vi "Configure Tone.vi"(0 "VISA resource name":refnum<visa-resource-name>, 1 "Frequency (1000 Hz)":dbl=1000.0, 2 "Phase (0 degrees)":dbl, 5 "Tone Channel (0: A)":i32(ring) items=["A", "B"], 7 "Tone Number (0)":i32, 9 "Amplitude (100 %)":dbl=100.0, 11 "error in (no error)":errorcluster, 12 "Enable Tone (T: Enable)":bool=TRUE) -> (4 "VISA resource name out":refnum<visa-resource-name>, 15 "error out":errorcluster)   [LabVIEW 2014, in "Stanford Research SR1.lvlib"]
doc: "Configures the attributes for the Tone."
uses:
  Stanford Research SR1.lvlib
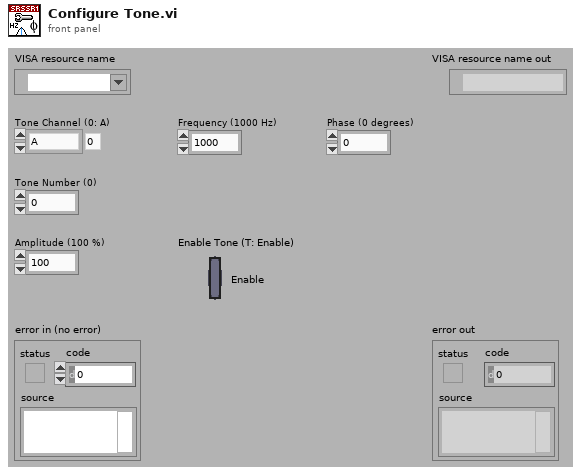
[diagram p1: front panel]
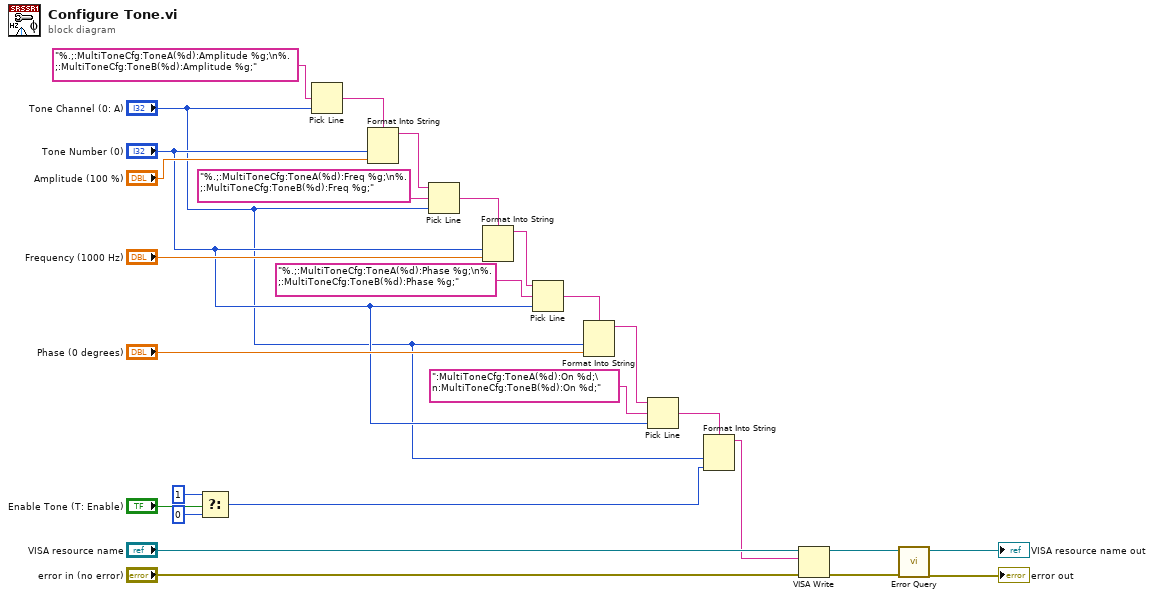
[diagram p0: block diagram]
diagram:
  n1 = Select(t=1, s="Enable Tone (T: Enable)", f=0) -> (s? t:f=w4:i32)
  n2 = Pick Line(multi-line string="%.;:MultiToneCfg:ToneA(%d):Amplitude %g;\n%.;:MultiToneCfg:ToneB(%d):Amplitude %g;", line index="Tone Channel (0: A)") -> (output string=w20:string)  [unwired: 1 in]
  n3 = Format Into String(format string=w20, "Tone Number (0)", "Amplitude (100 %)") -> (resulting string=w16:string)  [unwired: 2 in, 1 out]
  n4 = Pick Line(string ("")=w16, multi-line string="%.;:MultiToneCfg:ToneA(%d):Freq %g;\n%.;:MultiToneCfg:ToneB(%d):Freq %g;", line index="Tone Channel (0: A)") -> (output string=w18:string)
  n5 = Format Into String(format string=w18, "Tone Number (0)", "Frequency (1000 Hz)") -> (resulting string=w1:string)  [unwired: 2 in, 1 out]
  n6 = Pick Line(string ("")=w1, multi-line string="%.;:MultiToneCfg:ToneA(%d):Phase %g;\n%.;:MultiToneCfg:ToneB(%d):Phase %g;", line index="Tone Number (0)") -> (output string=w13:string)
  n7 = Format Into String(format string=w13, "Tone Channel (0: A)", "Phase (0 degrees)") -> (resulting string=w2:string)  [unwired: 2 in, 1 out]
  n8 = Pick Line(string ("")=w2, multi-line string=":MultiToneCfg:ToneA(%d):On %d;\n:MultiToneCfg:ToneB(%d):On %d;", line index="Tone Number (0)") -> (output string=w9:string)
  n9 = Format Into String(format string=w9, "Tone Channel (0: A)", w4) -> (resulting string=w3:string)  [unwired: 2 in, 1 out]
  n10 = VISA Write(VISA resource name="VISA resource name", write buffer=w3, error in (no error)="error in (no error)") -> (VISA resource name out=w25:refnum<visa-resource-name>, error out=w24:errorcluster)  [unwired: 1 out]
  n11 = call "Error Query.vi"("error in (no error)"=w24, "VISA resource name"=w25) -> ("error out"=→"error out":errorcluster, "VISA resource name out"=→"VISA resource name out":refnum<visa-resource-name>)  [unwired: 6 in, 2 out]
